vi "Calcula epoch.vi"() -> (0 "epoch":dbl format="%.11f")   [LabVIEW 2012]
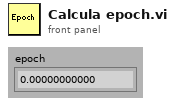
[diagram p1: front panel]
types:
  T1 = cluster{"second":i32, "minute":i32, "hour":i32, "day of month":i32, "month":i32, "year":i32, "day of week":i32, "day of year":i32, "is DST":i32}
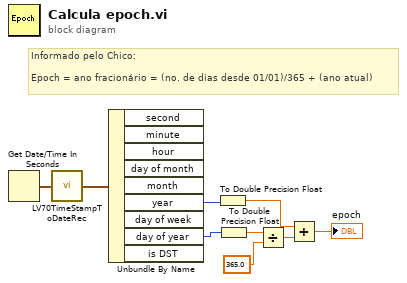
[diagram p0: block diagram]
diagram:
  # "Informado pelo Chico:\n\nEpoch = ano fracionário = (no. de dias desde 01/01)/365 + (ano atual)"
  n1 = Get Date/Time In Seconds() -> (seconds since 1Jan1904=w8:timestamp)
  n2 = call <vilib>:"LV70TimeStampToDateRec.vi"("time stamp"=w8) -> ("date time rec"=w9:T1)
  n3 = Unbundle By Name(w9) -> ("year"=w3:i32, "day of year"=w7:i32)  [unwired: 7 out]
  n4 = To Double Precision Float(number=w3) -> (double precision float=w2:dbl)
  n5 = To Double Precision Float(number=w7) -> (double precision float=w6:dbl)
  n6 = Divide(x=w6, y=365.0) -> (x/y=w4:dbl)
  n7 = Add(x=w2, y=w4) -> (x+y=→"epoch":dbl)
